vi "Paths_for_Seq_Shot.vi"(4 "File Path":T1={"Filename Prefix"="MyData", "Extension"=enum."±Field", "Suffix"="", "Current Path"=path "/opticsmac/Users/Data"}, 6 "FieldRamp Parameters":dbl[][](array[numeric])=[[0.0, 30.0, 1.0, 400.0], [30.0, 0.0, -1.0, 400.0], [0.0, -30.0, -1.0, 400.0], [-30.0, 0.0, 1.0, 400.0], [0.0, 30.0, 0.5, 200.0], [30.0, 0.0, -0.5, 200.0]] step=1.0 format="%.2f", 7 "RampIndexSelect":bool[](array[boolean])=[TRUE, TRUE, FALSE, FALSE, FALSE, FALSE]) -> (0 "File Path Para Array out":T1[](array[typedef]), 2 "FieldRamp Parameters out":dbl[][](array[numeric])=[[0.0, 30.0, 1.0, 400.0], [30.0, 0.0, -1.0, 400.0], [0.0, -30.0, -1.0, 400.0], [-30.0, 0.0, 1.0, 400.0], [0.0, 30.0, 0.5, 200.0], [30.0, 0.0, -0.5, 200.0]] step=1.0 format="%.2f", 3 "RampIndexSelect out":bool[](array[boolean])=[TRUE, TRUE, FALSE, FALSE, FALSE, FALSE])   [LabVIEW 2019]
uses:
  Globals and TypeDefs/Type Definitions.llb/FilePathParameter.ctt
panel:
  out "FilePrefix for the sequences":string[](array[string])
  in  "All Sequences":bool
  out "Default Path for the sequences":path[](array[path])
  in  "Go Ahead":bool
  in  "Diff Prefix?":bool=TRUE caption="Same Prefix"
  in  "FilePrefix":string[](array[string])=["", "", "", "", "", ""]
  in  "Sub Folder?":bool=TRUE caption="No Sub Folder"
  in  "SubfolderName":string[](array[string])=["", "", "", "", "", ""]
  # "Make sure that EVERYTHING is OK \nbefore proceeding to a series of\nCCD/InGaAs-PDA shots at specified \nmagnetic fields!\n\nYou can change some of the parameters here.\nIf you are unsure, click the Cancel button."
  # "Select   StartField (T)   EndField (T)   FieldStep (T)"
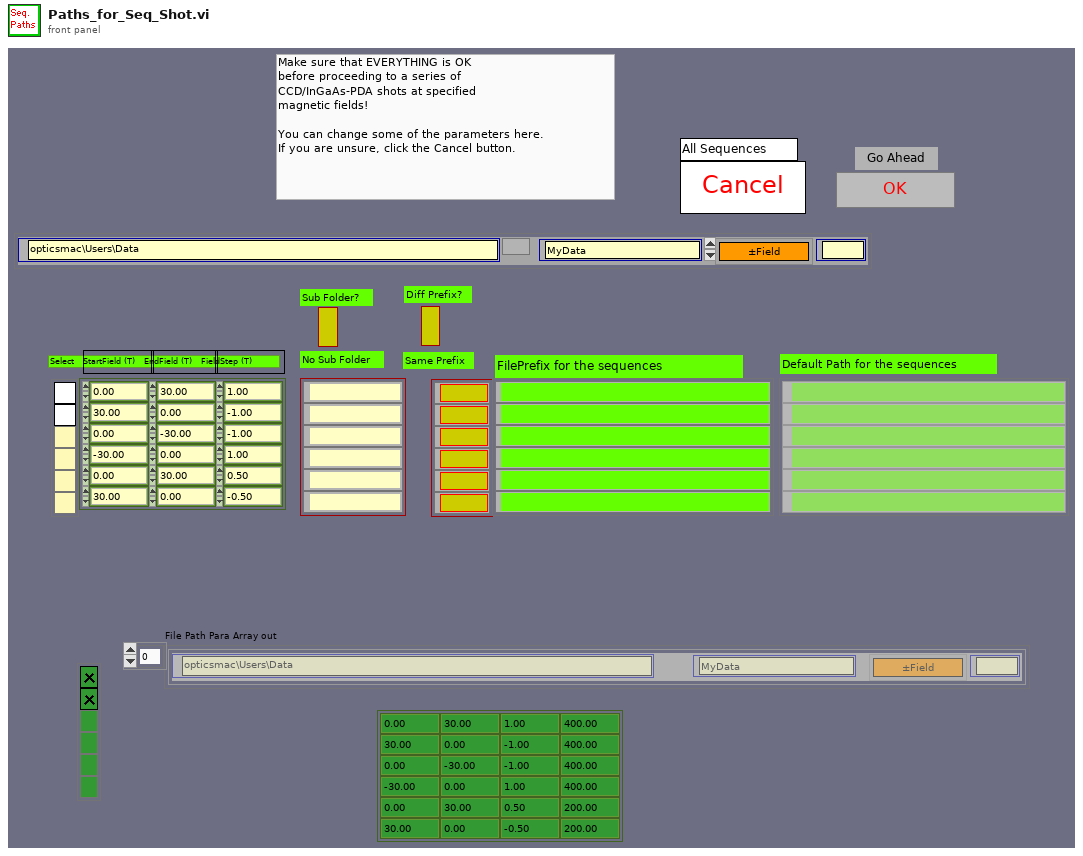
[diagram p1: front panel]
types:
  T1 = typedef "FilePathParameter.ctt" = cluster{"Filename Prefix":string, "Extension":enum16{"none", "\".001\",\".002\", ...", "001 (No dot)", "±Field", "pField nField", "Temperature", "Wavelength", "T(K)±H(T)", "(nm)T(K)±H(T)", "User Defined"}, "Suffix":string, "Current Path":path}
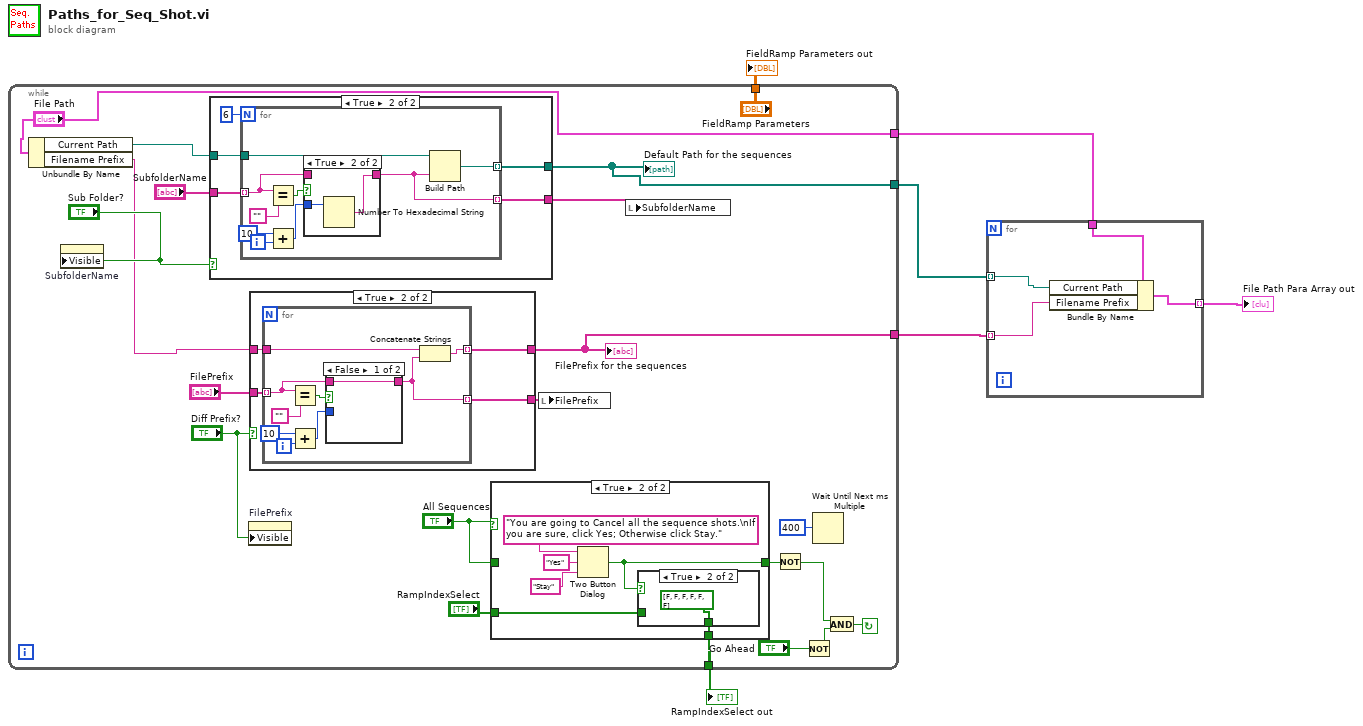
[diagram p0: block diagram]
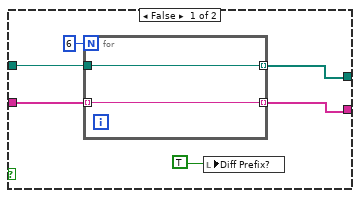
[diagram p2: hidden frame]
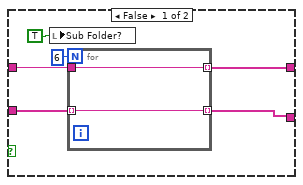
[diagram p4: hidden frame]
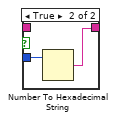
[diagram p5: hidden frame]
diagram:
  n1 = while {
    tunnel: [w26] -> w5
    tunnel: ["FieldRamp Parameters"] -> w6
    tunnel: [w11] -> w4
    tunnel: [w10] -> w3
    tunnel: ["File Path"] -> w2
    stop <- w21 continue-if-true
    n2 = Unbundle By Name("File Path") -> ("Current Path"=w12:path, "Filename Prefix"=w13:string)
    n3 = property on="SubfolderName" class="Arr (strict)"("Visible"="Sub Folder?") -> ()  [unwired: 2 in, 2 out]
    n4 = case shown="True" "Sub Folder?" {
      tunnel: "SubfolderName" -> [w29 w39]
      tunnel: w12 -> [w31 w38]
      tunnel: [w30 w37] -> w11
      tunnel: [w28 w36] -> w18
      frame False {
        n5 = for {
          N: 6 -> [_]
          tunnel: [w35] -> w30 mode=indexing
          tunnel: w31 -> [w35]
          tunnel: [w34] -> w28 mode=indexing
          tunnel: w29 -> [w34] mode=indexing
        }
        n6 = local write "Diff Prefix?"(TRUE ("Diff Prefix?")) -> ()
      }
      frame True {
        n7 = for {
          N: 6 -> [_]
          tunnel: w39 -> [w47] mode=indexing
          tunnel: w38 -> [w46]
          tunnel: [w45] -> w37 mode=indexing
          tunnel: [w42] -> w36 mode=indexing
          i -> [w44]
          n8 = Equal?(x=w47, y="") -> (x = y?=w48:bool)
          n9 = Add(x=10, y=w44) -> (x+y=w41:i32)
          n10 = case shown="True" w48 {
            tunnel: w47 -> [w50 _]
            tunnel: [w50 w51] -> w42
            tunnel: w41 -> [_ w52]
            frame False {
            }
            frame True {
              n11 = Number To Hexadecimal String(2:w52) -> (0:w51:string)  [unwired: 1 in]
            }
          }
          n12 = Build Path(base path=w46, name or relative path=w42) -> (appended path=w45:path)
        }
      }
    }
    "Default Path for the sequences" <- w11
    n13 = property on="FilePrefix" class="Arr (strict)"("Visible"="Diff Prefix?") -> ()  [unwired: 2 in, 2 out]
    n14 = case shown="True" "Diff Prefix?" {
      tunnel: w13 -> [w56 w62]
      tunnel: [w55 w61] -> w10
      tunnel: "FilePrefix" -> [w54 w64]
      tunnel: [w53 w63] -> w16
      frame False {
        n15 = local write "Sub Folder?"(TRUE ("Sub Folder?")) -> ()
        n16 = for {
          N: 6 -> [_]
          tunnel: w56 -> [w60]
          tunnel: [w60] -> w55 mode=indexing
          tunnel: w54 -> [w59] mode=indexing
          tunnel: [w59] -> w53 mode=indexing
        }
      }
      frame True {
        n17 = for {
          tunnel: w64 -> [w71] mode=indexing
          tunnel: [w66] -> w63 mode=indexing
          tunnel: w62 -> [w67]
          tunnel: [w65] -> w61 mode=indexing
          i -> [w70]
          n18 = Equal?(x=w71, y="") -> (x = y?=w72:bool)
          n19 = Add(x=10, y=w70) -> (x+y=w68:i32)
          n20 = case shown="False" w72 {
            tunnel: w71 -> [w74 _]
            tunnel: [w74 w75] -> w66
            tunnel: w68 -> [_ w76]
            frame False {
            }
            frame True {
              n21 = Number To Hexadecimal String(2:w76) -> (0:w75:string)  [unwired: 1 in]
            }
          }
          n22 = Concatenate Strings(w67, w66) -> (w65:string)
        }
      }
    }
    "FilePrefix for the sequences" <- w10
    n23 = case shown="True" "All Sequences" {
      tunnel: [w77 w81] -> w23
      tunnel: [w78 w80] -> w26
      tunnel: "RampIndexSelect" -> [w78 w79]
      tunnel: "All Sequences" -> [w77 _]
      frame False {
      }
      frame True {
        n24 = Two Button Dialog(message="You are going to Cancel all the sequence shots.\nIf you are sure, click Yes; Otherwise click Stay.", 1:"Stay" ("F button name (\"Cancel\")"), 2:"Yes" ("T button name (\"OK\")")) -> (T button?=w81:bool)
        n25 = case shown="True" w81 {
          tunnel: [w85 bool[] [FALSE, FALSE, FALSE, FALSE, FALSE, FALSE] ("RampIndexSelect out")] -> w80
          tunnel: w79 -> [w85 _]
          frame False {
          }
          frame True {
          }
        }
      }
    }
    n26 = local write "FilePrefix"(w16) -> ()
    n27 = local write "SubfolderName"(w18) -> ()
    n28 = Not(x=w23) -> (.not. x?=w22:bool)
    n29 = Not(x="Go Ahead") -> (.not. x?=w8:bool)
    n30 = Wait Until Next ms Multiple(millisecond multiple=u32 400) -> ()  [unwired: 1 out]
    n31 = And(x=w22, y=w8) -> (x .and. y?=w21:bool)
  }
  "FieldRamp Parameters out" <- w6
  "RampIndexSelect out" <- w5
  n32 = for {
    tunnel: w4 -> [w89] mode=indexing
    tunnel: w3 -> [w88] mode=indexing
    tunnel: w2 -> [w90]
    tunnel: [w87] -> w1 mode=indexing
    n33 = Bundle By Name(cluster=w90, "Current Path"=w89, "Filename Prefix"=w88) -> (w87:T1)
  }
  "File Path Para Array out" <- w1
